vi "FPGA_lock-in_analysis-light.vi"() -> ()   [LabVIEW 2013]
uses:
  <vilib>/LabVIEW Targets/FPGA/cRIO/shared/nicrio_ModuleControls/nicrio_cRIO-9205_VoltageRange.ctl
  <vilib>/rvi/Emulation/niFpgaSctlEmulationGetInTimedLoop.vi
  <vilib>/rvi/Emulation/niFpgaEmulationReportErrorSimple.vi
  <vilib>/rvi/Emulation/niFpgaGetClockAttributes.vi
  <vilib>/rvi/FIFO/Fifo_Resource/nirvififoEmulationReadFpgaImpl.vi
  <vilib>/rvi/DataTransferAndStorage/Container/Common/niFpgaContainerGetUniqueNameForEmu.vi
  <vilib>/rvi/Emulation/niFpgaProcessEmulError.vi
  <vilib>/rvi/Emulation/niFpgaCriticalErrorInLSC.vi
  <vilib>/rvi/eio/common/nirviEmuTemplateMethod_errors.vi
  <vilib>/rvi/FIFO/Fifo_Resource/nirvififoEmulationWriteFpgaImpl.vi
  <vilib>/rvi/interface/RandomDataEmulation/nirviRandomDataFPGAFIFO.vi
  <vilib>/rvi/interface/RandomDataEmulation/niFpgaRandomDataHandleErrors.vi
  <vilib>/rvi/DataTransferAndStorage/Container/XNode/niFpgaContainer.xnode
  <vilib>/rvi/FIFO/Fifo_Resource/nirvififoEmulationRead.vi
  <vilib>/eio/EIONode/EIONode.xnode
  <vilib>/rvi/FIFO/Fifo_Resource/nirvififoEmulationWrite.vi
  <vilib>/rvi/interface/RandomDataEmulation/nirviRandomDataFpgaReadWriteTemplate.vi
  <vilib>/eio/EIOMethodNode/EIOMethodNode.xnode
panel:
  in  "data-sent-to-host":enum8{"LI", "average"}(ring)
  in  "dt/tau":fxp<+,25,0>
  in  "Voltage Range":T1
  in  "lock-in input channel":u8 max=31 step=1
  out "XXX lock-in IN":fxp<+/-,26,5> format="%.23g"
  # "dt is the time between two points ( @ 250 kSample/s )"
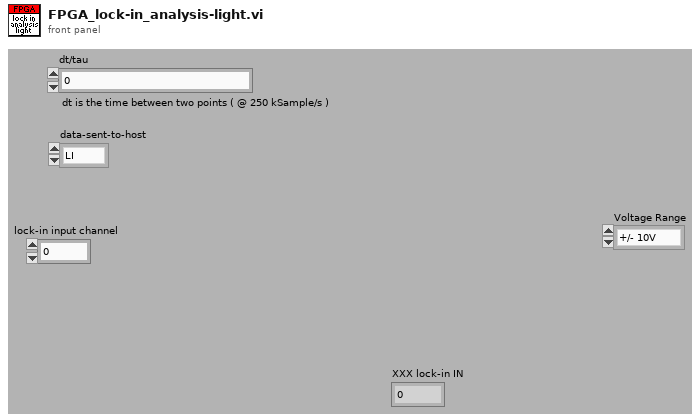
[diagram p1: front panel]
types:
  T1 = typedef "nicrio_cRIO-9205_VoltageRange.ctl" = enum8{"+/- 10V", "+/- 5V", "+/- 1V", "+/- 200mV"}
  T2 = cluster{"Boolean array[0]":bool, "Boolean array[1]":bool}
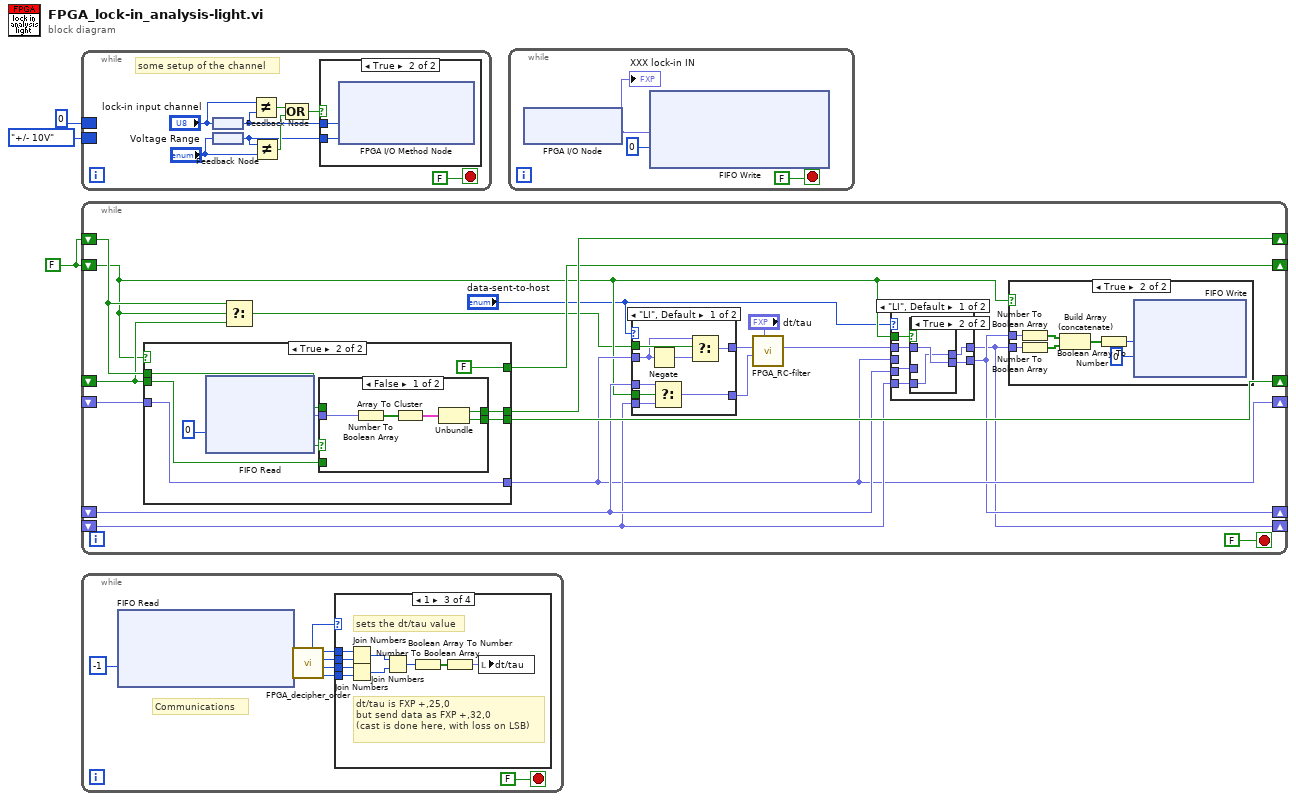
[diagram p0: block diagram]
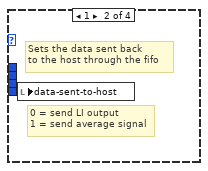
[diagram p3: hidden frame]
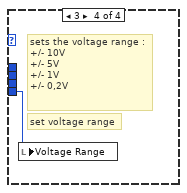
[diagram p4: hidden frame]
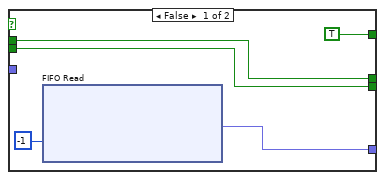
[diagram p10: hidden frame]
diagram:
  w1 = FALSE
  n1 = while {
    border: u8 0 ("AI Channel") -> [_]
    border: nicrio_cRIO-9205_VoltageRange."+/- 10V" ("Voltage Range") -> [_]
    stop <- FALSE stop-if-true
    # "some setup of the channel"
    n2 = feedback-in #1("lock-in input channel") -> ()
    n3 = feedback #1() -> (w10:u8)
    n4 = feedback-in #2("Voltage Range") -> ()
    n5 = feedback #2() -> (w5:T1)
    n6 = Not Equal?(x="lock-in input channel", y=w10) -> (x != y?=w8:bool)
    n7 = Not Equal?(x=w5, y="Voltage Range") -> (x != y?=w9:bool)
    n8 = Compound Arithmetic op=OR(w8, w9) -> (w7:bool)
    n9 = case shown="True" w7 {
      tunnel: w5 -> [_ w13]
      tunnel: w10 -> [_ w12]
      frame False {
      }
      frame True {
        n10 = xnode "FPGA I/O Method Node"("AI Channel"=w12, "Voltage Range"=w13) -> ()  [unwired: 1 in, 1 out]
      }
    }
  }
  n11 = while {
    shift-right: [w31] -> _
    shift-left: w1 -> [w26]
    shift-right: [w30] -> _
    shift-left: _ -> [w25]
    shift-right: [w18] -> _
    shift-left: _ -> [w22]
    shift-right: [w14] -> _
    shift-left: _ -> [w21]
    shift-right: [w27] -> _
    shift-left: w1 -> [w19]
    shift-right: [w20] -> _
    shift-left: _ -> [w16]
    stop <- FALSE stop-if-true
    n12 = case shown="False" w19 {
      tunnel: [w65 w72] -> w31
      tunnel: [w64 w71] -> w30
      tunnel: w25 -> [w64 w70]
      tunnel: w26 -> [w65 w69]
      tunnel: [w62 w67] -> w20
      tunnel: [TRUE FALSE] -> w27
      tunnel: w16 -> [_ w67]
      frame False {
        n13 = xnode ("FIFO Read")("Timeout"=-1) -> ("Element"=w62:fxp<+/-,26,5>)  [unwired: 1 in, 2 out]
      }
      frame True {
        n14 = xnode ("FIFO Read")("Timeout"=0) -> ("Element"=w73:fxp<+,2,2>, "Timed Out?"=w74:bool)  [unwired: 1 in, 1 out]
        n15 = case shown="False" w74 {
          tunnel: w73 -> [w80 _]
          tunnel: [w77 w82] -> w72
          tunnel: [w76 w81] -> w71
          tunnel: w69 -> [_ w82]
          tunnel: w70 -> [_ w81]
          frame False {
            n16 = Number To Boolean Array(number=w80) -> (Boolean array=w79:bool[])
            n17 = Array To Cluster(array=w79) -> (cluster=w78:T2)
            n18 = Unbundle(w78) -> ("Boolean array[0]"=w77:bool, "Boolean array[1]"=w76:bool)
          }
          frame True {
          }
        }
      }
    }
    n19 = Select(t=w26, s=w19, f=w25) -> (s? t:f=w15:bool)
    n20 = case shown="\"LI\", Default" "data-sent-to-host" {
      tunnel: [w52 w60] -> w29
      tunnel: w20 -> [w54 w60]
      tunnel: [w59 w61] -> w24
      tunnel: w19 -> [w58 _]
      tunnel: w22 -> [w57 _]
      tunnel: w21 -> [w56 w61]
      tunnel: w15 -> [w55 _]
      frame "LI", Default {
        n21 = Negate(x=w54) -> (-x=w53:fxp<+/-,27,6>)
        n22 = Select(t=w57, s=w58, f=w56) -> (s? t:f=w59:fxp<+/-,32,5>)
        n23 = Select(t=w54, s=w55, f=w53) -> (s? t:f=w52:fxp<+/-,27,6>)
      }
      frame "average" {
      }
    }
    n24 = call "FPGA_RC-filter.vi"("deltaT/tau"="dt/tau", "X_n"=w24, "mesure"=w29) -> ("X_n+1"=w23:fxp<+/-,32,5>)  [unwired: 8 out]
    n25 = case shown="\"LI\", Default" "data-sent-to-host" {
      tunnel: w19 -> [w45 _]
      tunnel: w23 -> [w44 w51]
      tunnel: [w43 w50] -> w18
      tunnel: [w42 w51] -> w14
      tunnel: w22 -> [w41 _]
      tunnel: w21 -> [w40 _]
      tunnel: w20 -> [_ w50]
      frame "LI", Default {
        n26 = case shown="True" w45 {
          tunnel: w44 -> [w47 w49]
          tunnel: [w46 w49] -> w43
          tunnel: [w47 w48] -> w42
          tunnel: w41 -> [w46 _]
          tunnel: w40 -> [_ w48]
          frame False {
          }
          frame True {
          }
        }
      }
      frame "average" {
      }
    }
    n27 = case shown="True" w19 {
      tunnel: w18 -> [_ w37]
      tunnel: w14 -> [_ w36]
      frame False {
      }
      frame True {
        n28 = Number To Boolean Array(number=w37) -> (Boolean array=w35:bool[])
        n29 = Number To Boolean Array(number=w36) -> (Boolean array=w34:bool[])
        n30 = Build Array (concatenate)(w35, w34) -> (w33:bool[])
        n31 = Boolean Array To Number(Boolean array=w33) -> (number=w38:u64)
        n32 = xnode ("FIFO Write")("Element"=w38, "Timeout"=0) -> ()  [unwired: 1 in, 2 out]
      }
    }
  }
  n33 = while {
    stop <- FALSE stop-if-true
    # "Communications"
    n34 = xnode ("FIFO Read")("Timeout"=-1) -> ("Element"=w88:u64)  [unwired: 1 in, 2 out]
    n35 = call "FPGA_decipher_order.vi"("order in"=w88) -> ("data 1"=w86:u8, "data 2"=w85:u8, "data 3"=w84:u8, "data 4"=w83:u8, "order out"=w87:u8)  [unwired: 6 out]
    n36 = case shown="1" w87 {
      tunnel: w86 -> [_ w91 w97 w101]
      tunnel: w85 -> [_ _ w98 _]
      tunnel: w84 -> [_ _ w99 _]
      tunnel: w83 -> [_ _ w100 _]
      frame 0, Default {
      }
      frame 1 {
        # "0 = send LI output\n1 = send average signal"
        # "Sets the data sent back \nto the host through the fifo"
        n37 = local write "data-sent-to-host"(w91) -> ()
      }
      frame 2 {
        # "dt/tau is FXP +,25,0\nbut send data as FXP +,32,0\n(cast is done here, with loss on LSB)"
        # "sets the dt/tau value"
        n38 = Join Numbers(hi=w100, lo=w99) -> ((hi.lo)=w95:u16)
        n39 = Join Numbers(hi=w98, lo=w97) -> ((hi.lo)=w96:u16)
        n40 = Join Numbers(hi=w95, lo=w96) -> ((hi.lo)=w94:u32)
        n41 = Number To Boolean Array(number=w94) -> (Boolean array=w93:bool[])
        n42 = Boolean Array To Number(Boolean array=w93) -> (number=w92:fxp<+/-,32,0>)
        n43 = local write "dt/tau"(w92) -> ()
      }
      frame 3 {
        # "sets the voltage range :\n+/- 10V\n+/- 5V\n+/- 1V\n+/- 0,2V"
        # "set voltage range"
        n44 = local write "Voltage Range"(w101) -> ()
      }
    }
  }
  n45 = while {
    stop <- FALSE stop-if-true
    n46 = xnode "FPGA I/O Node"() -> ("ModA/AI0"=w102:fxp<+/-,26,5>)  [unwired: 1 in, 1 out]
    "XXX lock-in IN" <- w102
    n47 = xnode ("FIFO Write")("Element"=w102, "Timeout"=0) -> ()  [unwired: 1 in, 2 out]
  }
